vi "Get Properties from Cluster.vi"(8 "error in":errorcluster, 10 "Variant Cluster":variant, 11 "custom device ref in":T1 format="%.0x") -> (0 "error out":errorcluster, 1 "Array":variant[](array[variant]), 2 "data":variant, 3 "custom device ref out":T1 format="%.0x")   [LabVIEW 2020, in "AIM ARINC 664 Scripting.lvlib"]
doc: "Be sure that cluster element names are matching Veristand Property names.\n\nDo not pass clusters of clusters or array of cluster as inputs to this VI. It only works with plain clusters."
uses:
  AIM ARINC 664 Scripting.lvlib
  <vilib>/NI VeriStand/Custom Device API/Custom Device Item Ref.ctl
  <vilib>/NI VeriStand/Custom Device API/Get Item Property (I32).vi
  <vilib>/NI VeriStand/Custom Device API/Get Item Property (Double).vi
  <vilib>/NI VeriStand/Custom Device API/Get Item Property (U32).vi
  <vilib>/NI VeriStand/Custom Device API/Get Item Property (U16).vi
  <vilib>/NI VeriStand/Custom Device API/Get Item Property (String).vi
  <vilib>/NI VeriStand/Custom Device API/Get Item Property (Path).vi
  <vilib>/NI VeriStand/Custom Device API/Get Item Property (Boolean).vi
  <vilib>/Utility/Data Type/NI_Data Type.lvlib
  <vilib>/NI VeriStand/Custom Device API/Custom Device API.lvlib
  <userlib>/_OpenG.lib/lvdata/lvdata.llb/openg_variant.lvlib
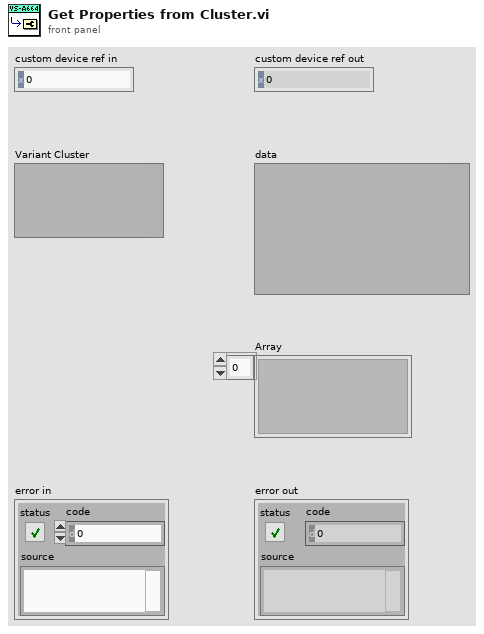
[diagram p1: front panel]
types:
  T1 = typedef "Custom Device API.lvlib/Custom Device Item Ref.ctl" = u64
  T2 = typedef "NI_Data Type.lvlib/Data Type.ctl" = enum8{"Invalid Type", "Void", "I8", "I16", "I32", "I64", "U8", "U16", "U32", "U64", "Single Float", "Double Float", "Extended Float", "Single Complex", "Double Complex", "Extended Complex", "Enum U8", "Enum U16", "Enum U32", "Enum U64", "Single Float With Unit", "Double Float With Unit", "Extended Float With Unit", "Single Complex with Unit", "Double Complex with Unit", "Extended Complex with Unit", "Boolean", "String", "Path", "Picture", "Tag", "Array", "Cluster", "Variant", "LV Variant", "Waveform", "Timestamp", "Digital Waveform", "Digital Data", "ExpressData", "Refnum", "External Data", "VI", "Poly VI", "LabVIEW Class Instance", "Fixed Point", "Set Collection", "Map Collection"}
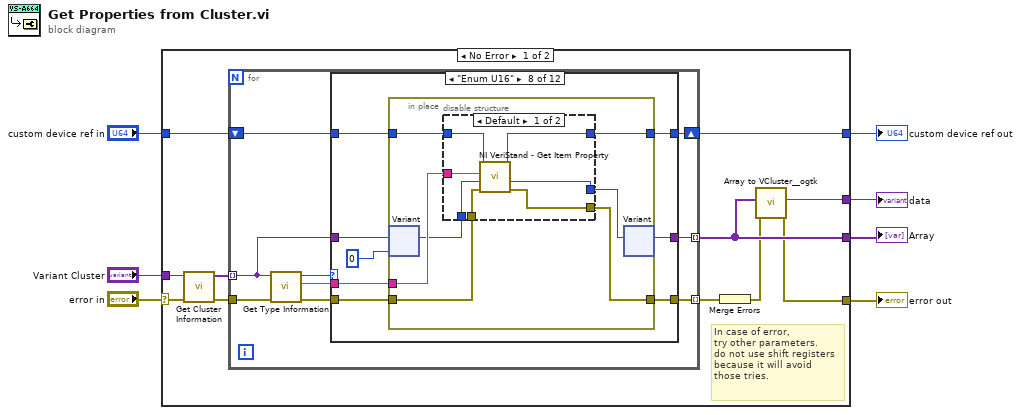
[diagram p0: block diagram]
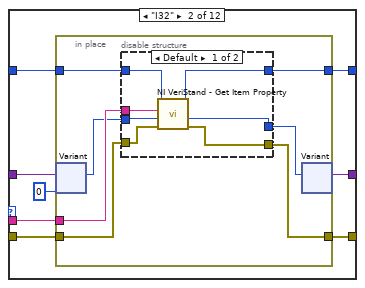
[diagram p3: hidden frame]
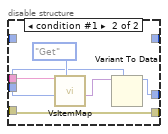
[diagram p4: hidden frame]
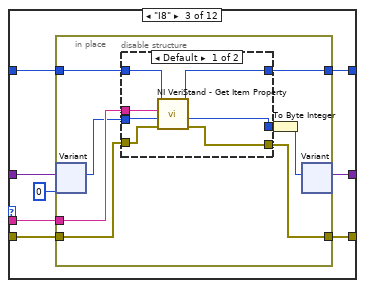
[diagram p5: hidden frame]
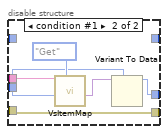
[diagram p6: hidden frame]
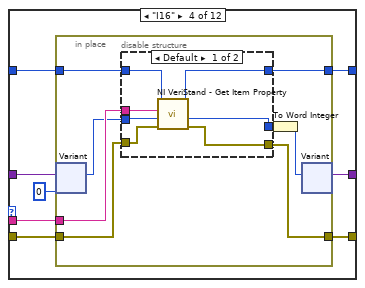
[diagram p7: hidden frame]
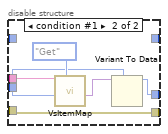
[diagram p8: hidden frame]
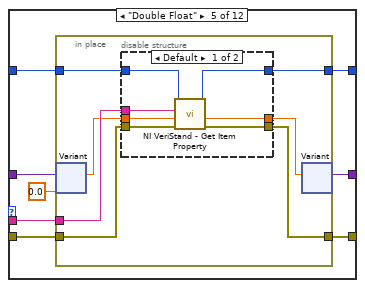
[diagram p9: hidden frame]
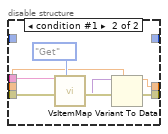
[diagram p10: hidden frame]
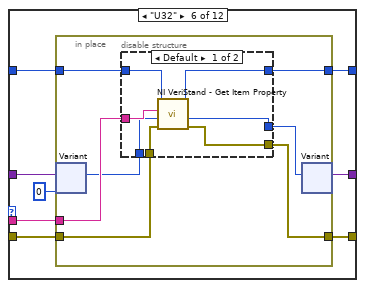
[diagram p11: hidden frame]
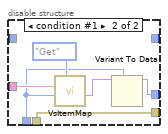
[diagram p12: hidden frame]
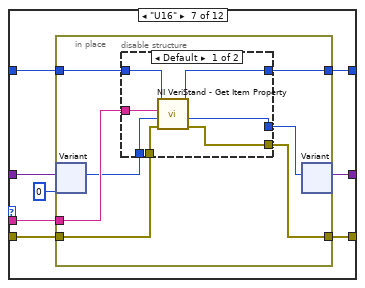
[diagram p13: hidden frame]
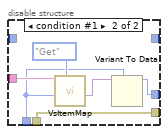
[diagram p14: hidden frame]
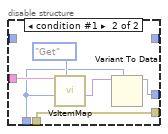
[diagram p15: hidden frame]
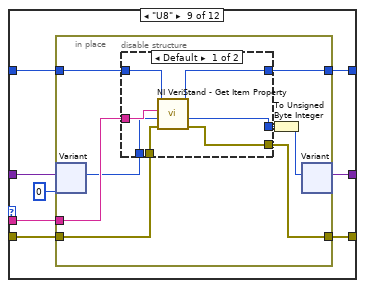
[diagram p16: hidden frame]
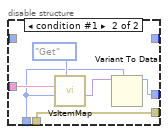
[diagram p17: hidden frame]
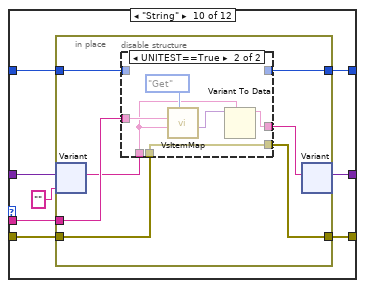
[diagram p18: hidden frame]
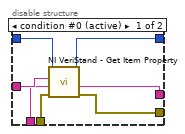
[diagram p19: hidden frame]
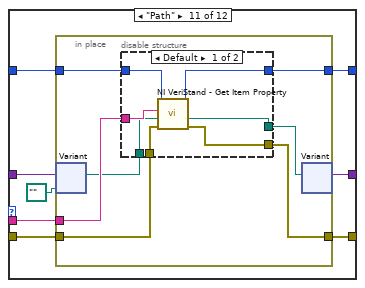
[diagram p20: hidden frame]
diagram:
  n1 = case shown="No Error" "error in" {
    selector: "error in" -> [w8 w343]
    tunnel: "custom device ref in" -> [w18 w342]
    tunnel: [w16 w342] -> w6
    tunnel: "Variant Cluster" -> [w13 _]
    tunnel: [w12 _] -> w4
    tunnel: [w11 _] -> w3
    tunnel: [w9 w343] -> w2
    frame No Error {
      # "In case of error,\ntry other parameters.\ndo not use shift registers\nbecause it will avoid \nthose tries."
      n2 = call <vilib>:"Get Cluster Information.vi"("error in (no error)"=w8, "variant"=w13) -> ("error out"=w14:errorcluster, "cluster elements"=w15:variant[])  [unwired: 8 in]
      n3 = for {
        tunnel: w15 -> [w20] mode=indexing
        shift-right: [w24] -> w16
        shift-left: w18 -> [w25]
        tunnel: [w21] -> w12 mode=indexing
        tunnel: w14 -> [w27]
        tunnel: [w19] -> w17 mode=indexing
        n4 = call <vilib>:"Get Type Information.vi"("error in (no error)"=w27, "variant"=w20) -> ("error out"=w22:errorcluster, "name"=w26:string, "type"=w23:T2)  [unwired: 5 in, 2 out]
        n5 = case shown="\"Enum U16\"" w23 {
          tunnel: w26 -> [_ w38 w66 w95 w124 w152 w180 w208 w236 w265 w293 w321]
          tunnel: w25 -> [w30 w37 w65 w94 w123 w151 w179 w207 w235 w264 w292 w320]
          tunnel: [w30 w36 w64 w93 w122 w150 w178 w206 w234 w263 w291 w319] -> w24
          tunnel: w22 -> [w29 w34 w62 w91 w120 w148 w176 w204 w232 w261 w289 w317]
          tunnel: [w29 w35 w63 w92 w121 w149 w177 w205 w233 w262 w290 w318] -> w19
          tunnel: w20 -> [w28 w33 w61 w90 w119 w147 w175 w203 w231 w260 w288 w316]
          tunnel: [w28 w32 w60 w89 w118 w146 w174 w202 w230 w259 w287 w315] -> w21
          frame "Invalid Type", Default {
          }
          frame "I32" {
            n6 = in-place {
              in-place-border: w38 -> [w45]
              in-place-border: w37 -> [w44]
              in-place-border: [w43] -> w36
              in-place-border: [w42] -> w35
              in-place-border: w34 -> [w41]
              n7 = in-place-variant #1(w33, 0) -> (w40:i32)  [unwired: 1 out]
              n8 = disable-structure shown="Default" {
                disable-tunnel: w45 -> [w52 w58]
                disable-tunnel: w44 -> [w51 _]
                disable-tunnel: [w50 _] -> w43
                disable-tunnel: [w49 w57] -> w42
                disable-tunnel: w40 -> [w48 w53]
                disable-tunnel: w41 -> [w47 w57]
                disable-tunnel: [w46 w55] -> w39
                frame condition #0 (active) {
                  n9 = call-poly <vilib>:"NI VeriStand - Get Item Property.vi"("error in (no error)"=w47, "Default Value"=w48, "Property Name"=w52, "Item Ref in"=w51) -> ("error out"=w49:errorcluster, "Value"=w46:i32, "Item Ref out"=w50:T1)  [unwired: 4 in, 1 out]
                }
                frame condition #1 {
                  n10 = call "VsItemMap.vi"("action (Set)"=enum16{"Set", "Get"}."Get", "Variant"=w53, "name"=w58) -> ("Variant out"=w54:variant)  [unwired: 8 in]
                  n11 = Variant To Data(type=w53, Variant=w54) -> (data=w55:i32)  [unwired: 1 in, 1 out]
                }
              }
              n12 = in-place-variant #1(w39) -> (w32:variant)  [unwired: 1 out]
            }
          }
          frame "I8" {
            n13 = in-place {
              in-place-border: w66 -> [w74]
              in-place-border: w65 -> [w73]
              in-place-border: [w72] -> w64
              in-place-border: [w71] -> w63
              in-place-border: w62 -> [w70]
              n14 = in-place-variant #2(w61, i8 0) -> (w69:i8)  [unwired: 1 out]
              n15 = disable-structure shown="Default" {
                disable-tunnel: w74 -> [w81 w87]
                disable-tunnel: w73 -> [w80 _]
                disable-tunnel: [w79 _] -> w72
                disable-tunnel: [w78 w86] -> w71
                disable-tunnel: w69 -> [w77 w82]
                disable-tunnel: w70 -> [w76 w86]
                disable-tunnel: [w75 w84] -> w68
                frame condition #0 (active) {
                  n16 = call-poly <vilib>:"NI VeriStand - Get Item Property.vi"("error in (no error)"=w76, "Default Value"=w77, "Property Name"=w81, "Item Ref in"=w80) -> ("error out"=w78:errorcluster, "Value"=w75:i32, "Item Ref out"=w79:T1)  [unwired: 4 in, 1 out]
                }
                frame condition #1 {
                  n17 = call "VsItemMap.vi"("action (Set)"=enum16{"Set", "Get"}."Get", "Variant"=w82, "name"=w87) -> ("Variant out"=w83:variant)  [unwired: 8 in]
                  n18 = Variant To Data(type=w82, Variant=w83) -> (data=w84:i8)  [unwired: 1 in, 1 out]
                }
              }
              n19 = To Byte Integer(number=w68) -> (8bit integer=w67:i8)
              n20 = in-place-variant #2(w67) -> (w60:variant)  [unwired: 1 out]
            }
          }
          frame "I16" {
            n21 = in-place {
              in-place-border: w95 -> [w103]
              in-place-border: w94 -> [w102]
              in-place-border: [w101] -> w93
              in-place-border: [w100] -> w92
              in-place-border: w91 -> [w99]
              n22 = in-place-variant #3(w90, i16 0) -> (w98:i16)  [unwired: 1 out]
              n23 = disable-structure shown="Default" {
                disable-tunnel: w103 -> [w110 w116]
                disable-tunnel: w102 -> [w109 _]
                disable-tunnel: [w108 _] -> w101
                disable-tunnel: [w107 w115] -> w100
                disable-tunnel: w98 -> [w106 w111]
                disable-tunnel: w99 -> [w105 w115]
                disable-tunnel: [w104 w113] -> w97
                frame condition #0 (active) {
                  n24 = call-poly <vilib>:"NI VeriStand - Get Item Property.vi"("error in (no error)"=w105, "Default Value"=w106, "Property Name"=w110, "Item Ref in"=w109) -> ("error out"=w107:errorcluster, "Value"=w104:i32, "Item Ref out"=w108:T1)  [unwired: 4 in, 1 out]
                }
                frame condition #1 {
                  n25 = call "VsItemMap.vi"("action (Set)"=enum16{"Set", "Get"}."Get", "Variant"=w111, "name"=w116) -> ("Variant out"=w112:variant)  [unwired: 8 in]
                  n26 = Variant To Data(type=w111, Variant=w112) -> (data=w113:i16)  [unwired: 1 in, 1 out]
                }
              }
              n27 = To Word Integer(number=w97) -> (16bit integer=w96:i16)
              n28 = in-place-variant #3(w96) -> (w89:variant)  [unwired: 1 out]
            }
          }
          frame "Double Float" {
            n29 = in-place {
              in-place-border: w124 -> [w131]
              in-place-border: w123 -> [w130]
              in-place-border: [w129] -> w122
              in-place-border: [w128] -> w121
              in-place-border: w120 -> [w127]
              n30 = in-place-variant #4(w119, 0.0) -> (w126:dbl)  [unwired: 1 out]
              n31 = disable-structure shown="Default" {
                disable-tunnel: w131 -> [w138 w144]
                disable-tunnel: w130 -> [w137 _]
                disable-tunnel: [w136 _] -> w129
                disable-tunnel: [w135 w143] -> w128
                disable-tunnel: w126 -> [w134 w139]
                disable-tunnel: w127 -> [w133 w143]
                disable-tunnel: [w132 w141] -> w125
                frame condition #0 (active) {
                  n32 = call-poly <vilib>:"NI VeriStand - Get Item Property.vi"("error in (no error)"=w133, "Default Value"=w134, "Property Name"=w138, "Item Ref in"=w137) -> ("error out"=w135:errorcluster, "Value"=w132:dbl, "Item Ref out"=w136:T1)  [unwired: 4 in, 1 out]
                }
                frame condition #1 {
                  n33 = call "VsItemMap.vi"("action (Set)"=enum16{"Set", "Get"}."Get", "Variant"=w139, "name"=w144) -> ("Variant out"=w140:variant)  [unwired: 8 in]
                  n34 = Variant To Data(type=w139, Variant=w140) -> (data=w141:dbl)  [unwired: 1 in, 1 out]
                }
              }
              n35 = in-place-variant #4(w125) -> (w118:variant)  [unwired: 1 out]
            }
          }
          frame "U32" {
            n36 = in-place {
              in-place-border: w152 -> [w159]
              in-place-border: w151 -> [w158]
              in-place-border: [w157] -> w150
              in-place-border: [w156] -> w149
              in-place-border: w148 -> [w155]
              n37 = in-place-variant #5(w147, u32 0) -> (w154:u32)  [unwired: 1 out]
              n38 = disable-structure shown="Default" {
                disable-tunnel: w159 -> [w166 w172]
                disable-tunnel: w158 -> [w165 _]
                disable-tunnel: [w164 _] -> w157
                disable-tunnel: [w163 w171] -> w156
                disable-tunnel: w154 -> [w162 w167]
                disable-tunnel: w155 -> [w161 w171]
                disable-tunnel: [w160 w169] -> w153
                frame condition #0 (active) {
                  n39 = call-poly <vilib>:"NI VeriStand - Get Item Property.vi"("error in (no error)"=w161, "Default Value"=w162, "Property Name"=w166, "Item Ref in"=w165) -> ("error out"=w163:errorcluster, "Value"=w160:u32, "Item Ref out"=w164:T1)  [unwired: 4 in, 1 out]
                }
                frame condition #1 {
                  n40 = call "VsItemMap.vi"("action (Set)"=enum16{"Set", "Get"}."Get", "Variant"=w167, "name"=w172) -> ("Variant out"=w168:variant)  [unwired: 8 in]
                  n41 = Variant To Data(type=w167, Variant=w168) -> (data=w169:u32)  [unwired: 1 in, 1 out]
                }
              }
              n42 = in-place-variant #5(w153) -> (w146:variant)  [unwired: 1 out]
            }
          }
          frame "U16" {
            n43 = in-place {
              in-place-border: w180 -> [w187]
              in-place-border: w179 -> [w186]
              in-place-border: [w185] -> w178
              in-place-border: [w184] -> w177
              in-place-border: w176 -> [w183]
              n44 = in-place-variant #6(w175, u16 0) -> (w182:u16)  [unwired: 1 out]
              n45 = disable-structure shown="Default" {
                disable-tunnel: w187 -> [w194 w200]
                disable-tunnel: w186 -> [w193 _]
                disable-tunnel: [w192 _] -> w185
                disable-tunnel: [w191 w199] -> w184
                disable-tunnel: w182 -> [w190 w195]
                disable-tunnel: w183 -> [w189 w199]
                disable-tunnel: [w188 w197] -> w181
                frame condition #0 (active) {
                  n46 = call-poly <vilib>:"NI VeriStand - Get Item Property.vi"("error in (no error)"=w189, "Default Value"=w190, "Property Name"=w194, "Item Ref in"=w193) -> ("error out"=w191:errorcluster, "Value"=w188:u16, "Item Ref out"=w192:T1)  [unwired: 4 in, 1 out]
                }
                frame condition #1 {
                  n47 = call "VsItemMap.vi"("action (Set)"=enum16{"Set", "Get"}."Get", "Variant"=w195, "name"=w200) -> ("Variant out"=w196:variant)  [unwired: 8 in]
                  n48 = Variant To Data(type=w195, Variant=w196) -> (data=w197:u16)  [unwired: 1 in, 1 out]
                }
              }
              n49 = in-place-variant #6(w181) -> (w174:variant)  [unwired: 1 out]
            }
          }
          frame "Enum U16" {
            n50 = in-place {
              in-place-border: w208 -> [w215]
              in-place-border: w207 -> [w214]
              in-place-border: [w213] -> w206
              in-place-border: [w212] -> w205
              in-place-border: w204 -> [w211]
              n51 = in-place-variant #7(w203, u16 0) -> (w210:u16)  [unwired: 1 out]
              n52 = disable-structure shown="Default" {
                disable-tunnel: w215 -> [w222 w228]
                disable-tunnel: w214 -> [w221 _]
                disable-tunnel: [w220 _] -> w213
                disable-tunnel: [w219 w227] -> w212
                disable-tunnel: w210 -> [w218 w223]
                disable-tunnel: w211 -> [w217 w227]
                disable-tunnel: [w216 w225] -> w209
                frame condition #0 (active) {
                  n53 = call-poly <vilib>:"NI VeriStand - Get Item Property.vi"("error in (no error)"=w217, "Default Value"=w218, "Property Name"=w222, "Item Ref in"=w221) -> ("error out"=w219:errorcluster, "Value"=w216:u16, "Item Ref out"=w220:T1)  [unwired: 4 in, 1 out]
                }
                frame condition #1 {
                  n54 = call "VsItemMap.vi"("action (Set)"=enum16{"Set", "Get"}."Get", "Variant"=w223, "name"=w228) -> ("Variant out"=w224:variant)  [unwired: 8 in]
                  n55 = Variant To Data(type=w223, Variant=w224) -> (data=w225:u16)  [unwired: 1 in, 1 out]
                }
              }
              n56 = in-place-variant #7(w209) -> (w202:variant)  [unwired: 1 out]
            }
          }
          frame "U8" {
            n57 = in-place {
              in-place-border: w236 -> [w244]
              in-place-border: w235 -> [w243]
              in-place-border: [w242] -> w234
              in-place-border: [w241] -> w233
              in-place-border: w232 -> [w240]
              n58 = in-place-variant #8(w231, u8 0) -> (w239:u8)  [unwired: 1 out]
              n59 = disable-structure shown="Default" {
                disable-tunnel: w244 -> [w251 w257]
                disable-tunnel: w243 -> [w250 _]
                disable-tunnel: [w249 _] -> w242
                disable-tunnel: [w248 w256] -> w241
                disable-tunnel: w239 -> [w247 w252]
                disable-tunnel: w240 -> [w246 w256]
                disable-tunnel: [w245 w254] -> w238
                frame condition #0 (active) {
                  n60 = call-poly <vilib>:"NI VeriStand - Get Item Property.vi"("error in (no error)"=w246, "Default Value"=w247, "Property Name"=w251, "Item Ref in"=w250) -> ("error out"=w248:errorcluster, "Value"=w245:u16, "Item Ref out"=w249:T1)  [unwired: 4 in, 1 out]
                }
                frame condition #1 {
                  n61 = call "VsItemMap.vi"("action (Set)"=enum16{"Set", "Get"}."Get", "Variant"=w252, "name"=w257) -> ("Variant out"=w253:variant)  [unwired: 8 in]
                  n62 = Variant To Data(type=w252, Variant=w253) -> (data=w254:u8)  [unwired: 1 in, 1 out]
                }
              }
              n63 = To Unsigned Byte Integer(number=w238) -> (unsigned 8bit integer=w237:u8)
              n64 = in-place-variant #8(w237) -> (w230:variant)  [unwired: 1 out]
            }
          }
          frame "String" {
            n65 = in-place {
              in-place-border: w265 -> [w272]
              in-place-border: w264 -> [w271]
              in-place-border: [w270] -> w263
              in-place-border: [w269] -> w262
              in-place-border: w261 -> [w268]
              n66 = in-place-variant #9(w260, "") -> (w267:string)  [unwired: 1 out]
              n67 = disable-structure shown="UNITEST==True" {
                disable-tunnel: w272 -> [w279 w285]
                disable-tunnel: w271 -> [w278 _]
                disable-tunnel: [w277 _] -> w270
                disable-tunnel: [w276 w284] -> w269
                disable-tunnel: w267 -> [w275 w280]
                disable-tunnel: w268 -> [w274 w284]
                disable-tunnel: [w273 w282] -> w266
                frame condition #0 (active) {
                  n68 = call-poly <vilib>:"NI VeriStand - Get Item Property.vi"("error in (no error)"=w274, "Default Value"=w275, "Property Name"=w279, "Item Ref in"=w278) -> ("error out"=w276:errorcluster, "Value"=w273:string, "Item Ref out"=w277:T1)  [unwired: 4 in, 1 out]
                }
                frame condition #1 {
                  n69 = call "VsItemMap.vi"("action (Set)"=enum16{"Set", "Get"}."Get", "Variant"=w280, "name"=w285) -> ("Variant out"=w281:variant)  [unwired: 8 in]
                  n70 = Variant To Data(type=w280, Variant=w281) -> (data=w282:string)  [unwired: 1 in, 1 out]
                }
              }
              n71 = in-place-variant #9(w266) -> (w259:variant)  [unwired: 1 out]
            }
          }
          frame "Path" {
            n72 = in-place {
              in-place-border: w293 -> [w300]
              in-place-border: w292 -> [w299]
              in-place-border: [w298] -> w291
              in-place-border: [w297] -> w290
              in-place-border: w289 -> [w296]
              n73 = in-place-variant #10(w288, path "") -> (w295:path)  [unwired: 1 out]
              n74 = disable-structure shown="Default" {
                disable-tunnel: w300 -> [w307 w313]
                disable-tunnel: w299 -> [w306 _]
                disable-tunnel: [w305 _] -> w298
                disable-tunnel: [w304 w312] -> w297
                disable-tunnel: w295 -> [w303 w308]
                disable-tunnel: w296 -> [w302 w312]
                disable-tunnel: [w301 w310] -> w294
                frame condition #0 (active) {
                  n75 = call-poly <vilib>:"NI VeriStand - Get Item Property.vi"("error in (no error)"=w302, "Default Value"=w303, "Property Name"=w307, "Item Ref in"=w306) -> ("error out"=w304:errorcluster, "Value"=w301:path, "Item Ref out"=w305:T1)  [unwired: 4 in, 1 out]
                }
                frame condition #1 {
                  n76 = call "VsItemMap.vi"("action (Set)"=enum16{"Set", "Get"}."Get", "Variant"=w308, "name"=w313) -> ("Variant out"=w309:variant)  [unwired: 8 in]
                  n77 = Variant To Data(type=w308, Variant=w309) -> (data=w310:path)  [unwired: 1 in, 1 out]
                }
              }
              n78 = in-place-variant #10(w294) -> (w287:variant)  [unwired: 1 out]
            }
          }
          frame "Boolean" {
            n79 = in-place {
              in-place-border: w321 -> [w328]
              in-place-border: w320 -> [w327]
              in-place-border: [w326] -> w319
              in-place-border: [w325] -> w318
              in-place-border: w317 -> [w324]
              n80 = in-place-variant #11(w316, FALSE) -> (w323:bool)  [unwired: 1 out]
              n81 = disable-structure shown="Default" {
                disable-tunnel: w328 -> [w335 w341]
                disable-tunnel: w327 -> [w334 _]
                disable-tunnel: [w333 _] -> w326
                disable-tunnel: [w332 w340] -> w325
                disable-tunnel: w323 -> [w331 w336]
                disable-tunnel: w324 -> [w330 w340]
                disable-tunnel: [w329 w338] -> w322
                frame condition #0 (active) {
                  n82 = call-poly <vilib>:"NI VeriStand - Get Item Property.vi"("error in (no error)"=w330, "Default Value"=w331, "Property Name"=w335, "Item Ref in"=w334) -> ("error out"=w332:errorcluster, "Value"=w329:bool, "Item Ref out"=w333:T1)  [unwired: 4 in, 1 out]
                }
                frame condition #1 {
                  n83 = call "VsItemMap.vi"("action (Set)"=enum16{"Set", "Get"}."Get", "Variant"=w336, "name"=w341) -> ("Variant out"=w337:variant)  [unwired: 8 in]
                  n84 = Variant To Data(type=w336, Variant=w337) -> (data=w338:bool)  [unwired: 1 in, 1 out]
                }
              }
              n85 = in-place-variant #11(w322) -> (w315:variant)  [unwired: 1 out]
            }
          }
        }
      }
      n86 = Merge Errors(w17) -> (w10:errorcluster)
      n87 = call <userlib>:"Array to VCluster__ogtk.vi"("error in (no error)"=w10, "Array"=w12) -> ("error out"=w9:errorcluster, "VCluster"=w11:variant)  [unwired: 8 in]
    }
    frame Error {
      # "In case of error in, bypass anything inside"
    }
  }
  "error out" <- w2
  "custom device ref out" <- w6
  "data" <- w3
  "Array" <- w4
